vi "incrementaAmplitud.vi"(0 "Señal de Control IN":dbl[](array[numeric]), 5 "Sound Parameters":cluster{"# samples":u32, "tiempos (ms)":dbl}, 7 "Parametros Actuales IN":T1, 9 "detla Parametros":T1, 11 "Parametros Maximos":T1) -> (4 "Out":dbl[](array[numeric]), 6 "Tope?":bool, 8 "Parametros Actuales OUT":T1)   [LabVIEW 2010]
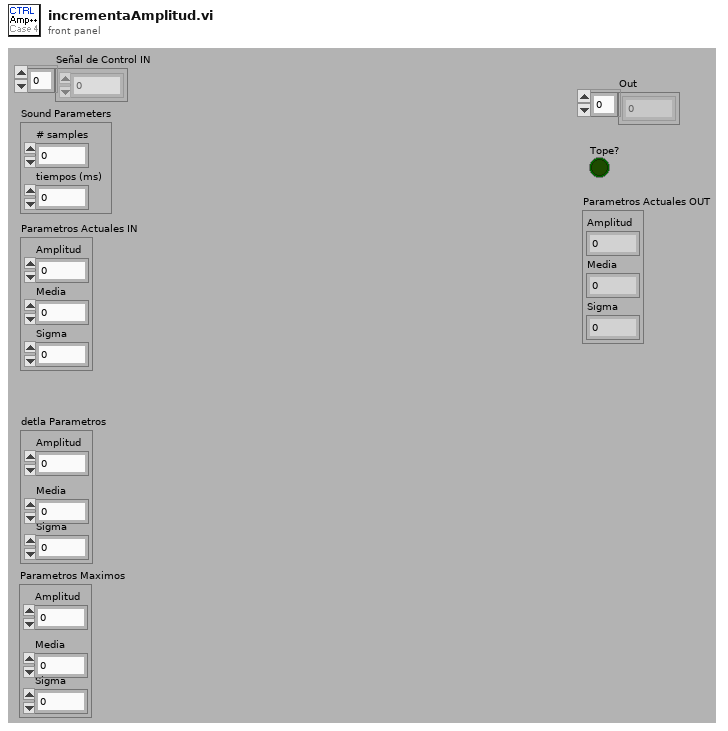
[diagram p1: front panel]
types:
  T1 = cluster{"Amplitud":dbl, "Media":dbl, "Sigma":dbl}
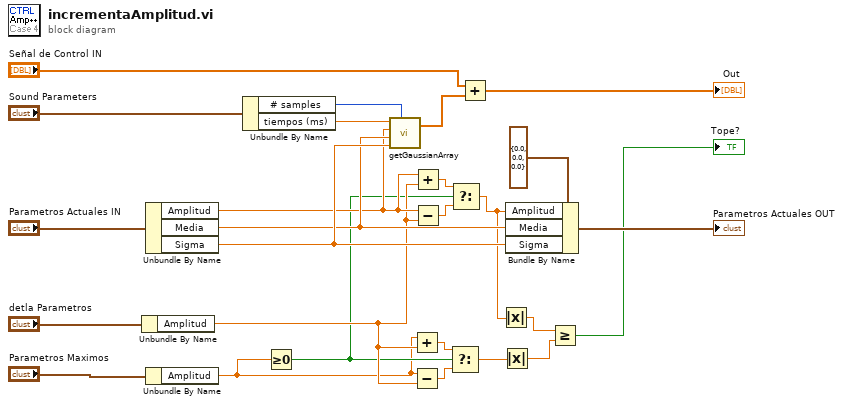
[diagram p0: block diagram]
diagram:
  n1 = Unbundle By Name("detla Parametros") -> ("Amplitud"=w7:dbl)
  n2 = Unbundle By Name("Parametros Actuales IN") -> ("Amplitud"=w12:dbl, "Media"=w13:dbl, "Sigma"=w14:dbl)
  n3 = Unbundle By Name("Parametros Maximos") -> ("Amplitud"=w1:dbl)
  n4 = Unbundle By Name("Sound Parameters") -> ("# samples"=w19:u32, "tiempos (ms)"=w18:dbl)
  n5 = Greater Or Equal To 0?(x=w1) -> (x >= 0?=w6:bool)
  n6 = call "getGaussianArray.vi"("tiempo (ms)"=w18, "Amplitud"=w12, "t0 (ms)"=w13, "Sigma (ms)"=w14, "#samples"=w19) -> ("Y out"=w25:dbl[])  [unwired: 1 out]
  n7 = Add(x=w1, y=w7) -> (x+y=w9:dbl)
  n8 = Subtract(x=w1, y=w7) -> (x-y=w8:dbl)
  n9 = Add(x=w12, y=w7) -> (x+y=w11:dbl)
  n10 = Subtract(x=w12, y=w7) -> (x-y=w10:dbl)
  n11 = Select(t=w9, s=w6, f=w8) -> (s? t:f=w4:dbl)
  n12 = Select(t=w11, s=w6, f=w10) -> (s? t:f=w5:dbl)
  n13 = Add(x="Señal de Control IN", y=w25) -> (x+y=→"Out":dbl[])
  n14 = Absolute Value(x=w5) -> (abs(x)=w3:dbl)
  n15 = Absolute Value(x=w4) -> (abs(x)=w2:dbl)
  n16 = Bundle By Name(cluster=T1 {"Amplitud"=0.0, "Media"=0.0, "Sigma"=0.0} ("input cluster"), "Amplitud"=w5, "Media"=w13, "Sigma"=w14) -> (→"Parametros Actuales OUT":T1)
  n17 = Greater Or Equal?(x=w3, y=w2) -> (x >= y?=→"Tope?":bool)
